vi "Write States.vi"(8 "error in (no error)":errorcluster, 10 "States":enum16{"Position", "Exit"}(ring), 11 "5RobotsTactic in":refnum<class "5RobotsTactic.lvclass">) -> (0 "error out":errorcluster, 3 "5RobotsTactic out":refnum<class "5RobotsTactic.lvclass">)   [LabVIEW 2020, in "5RobotsTactic.lvclass"]
uses:
  5RobotsTactic.lvclass
  5RobotsTactic.lvclass/5RobotsTactic.ctl
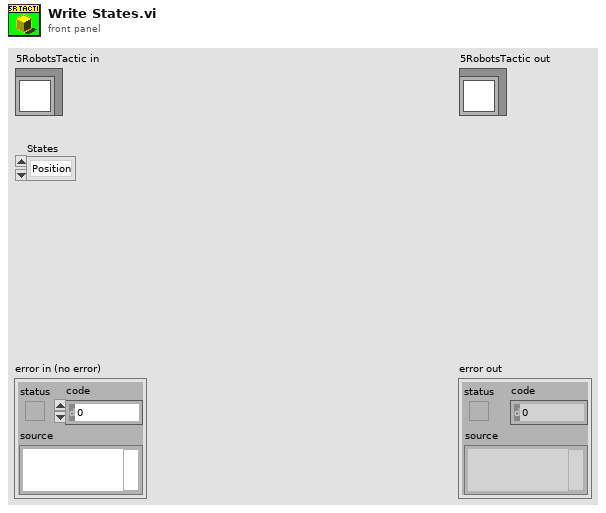
[diagram p1: front panel]
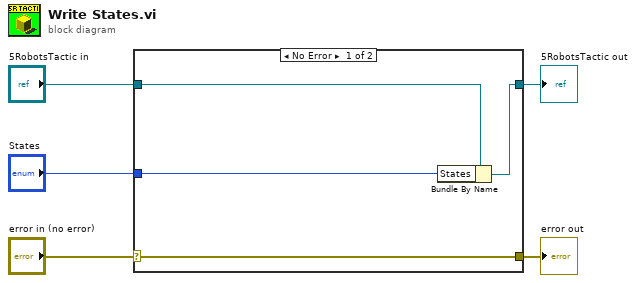
[diagram p0: block diagram]
diagram:
  n1 = case shown="No Error" "error in (no error)" {
    selector: "error in (no error)" -> [w9 w10]
    tunnel: [w9 w10] -> w4
    tunnel: [w7 w11] -> w2
    tunnel: "5RobotsTactic in" -> [w8 w11]
    tunnel: "States" -> [w6 _]
    frame No Error {
      n2 = Bundle By Name(cluster=w8, "States"=w6) -> (w7:refnum<class "5RobotsTactic.lvclass">)
    }
    frame Error {
    }
  }
  "error out" <- w4
  "5RobotsTactic out" <- w2
